vi "Enable Tap Channels.vi"(0 "fpga interface in":refnum<k20>, 5 "serial input channels":string[](array[string]), 11 "error in (no error)":errorcluster) -> (4 "fpga interface out":refnum<k20>, 15 "error out":errorcluster)   [LabVIEW 2023, in "GettingStarted_Tap_148X_Host.lvlib"]
uses:
  GettingStarted_Tap_148X_Host.lvlib
  Acq/Types/148x_Acq_FPGA_Reference.ctl
  <vilib>/Utility/error.llb/Error Cluster From Error Code.vi
  <vilib>/rvi/errors/niLvFpgaAdjustHostInterfaceError.vi
  <vilib>/rvi/interface/nirviReadWriteControl/nirviReadWriteControl.xnode
  Acq/GettingStarted_Acq_148X_Host.lvlib
  <vilib>/rvi/interface/Simulation/niFpgaSimulationCallBeginRW.vi
  NiFpgaLv.dll
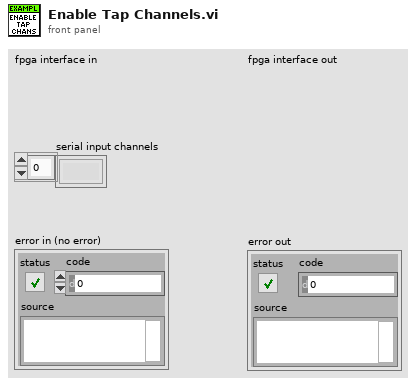
[diagram p1: front panel]
types:
  T1 = typedef "GettingStarted_Acq_148X_Host.lvlib/148x_Acq_FPGA_Reference.ctl" = refnum<k20>
  T2 = cluster{"channel acq config":cluster{"stop timeout (cycles)":u32, "first packet data type select mask":u64, "last packet data type select mask":u64, "first and last packet virtual channel must match":bool}, "virtual channel packet filter mask":u16, "data type packet filter mask":u64, "select corrected csi-2 data":bool, "enable channel":bool}[]
  T3 = cluster{"channel acq config":cluster{"stop timeout (cycles)":u32, "first packet data type select mask":u64, "last packet data type select mask":u64, "first and last packet virtual channel must match":bool}, "virtual channel packet filter mask":u16, "data type packet filter mask":u64, "select corrected csi-2 data":bool, "enable channel":bool}
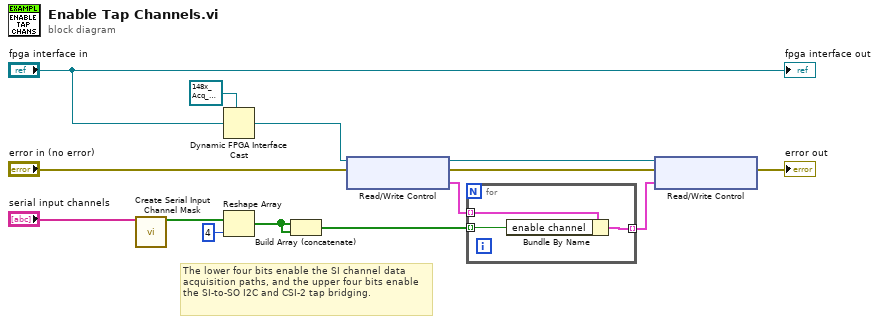
[diagram p0: block diagram]
diagram:
  # "The lower four bits enable the SI channel data acquisition paths, and the upper four bits enable the SI-to-SO I2C and CSI-2 tap bridging."
  n1 = call "Create Serial Input Channel Mask.vi"("serial channels"="serial input channels") -> ("serial input channel mask"=w2:bool[])  [unwired: 14 in]
  n2 = Dynamic FPGA Interface Cast(Session In=T1 refnum ("FPGA VI Reference Out"), Type="fpga interface in") -> (Session Out=w3:T1)
  n3 = Reshape Array(w2, 4 ("dimension size")) -> (w10:bool[])
  n4 = Build Array (concatenate)(w10, w10) -> (w5:bool[])
  n5 = xnode "Read/Write Control"("FPGA VI Reference In"=w3, "error in"="error in (no error)") -> ("FPGA VI Reference Out"=w7:T1, "error out"=w8:errorcluster, "channel configs"=w9:T2)
  n6 = for {
    tunnel: w9 -> [w17] mode=indexing
    tunnel: w5 -> [w16] mode=indexing
    tunnel: [w15] -> w6 mode=indexing
    n7 = Bundle By Name(cluster=w17, "enable channel"=w16) -> (w15:T3)
  }
  n8 = xnode "Read/Write Control"("FPGA VI Reference In"=w7, "error in"=w8, "channel configs"=w6) -> ("error out"=→"error out":errorcluster)  [unwired: 1 out]
  "fpga interface out" <- "fpga interface in"
